vi "XXPathPlanner_ConstraintsZone_IsWithinZone.vi"(9 "T":dbl, 11 "ConstraintsZone":T1={"minPosition"=0.0, "maxPosition"=0.0, "Constraints"={"MaxVelocityMps;"=0.0, "MaxAccelerationMpsSq;"=0.0, "MaxAngularVelRadPsEc;"=0.0, "MaxAngularAccRadPSecSq"=0.0, "Exists"=FALSE, "Unlimited"=FALSE, "NominalVoltageVolts"=12.0}, "Present"=FALSE}) -> (3 "WithinZone":bool)   [LabVIEW 2019]
doc: "Get if a given waypoint relative position is within this zone\n \nInputs:\n -- ConstraintsZone -- cluster -- data structure containing zone definition. \n -- t - double - Waypoint relative position\n\nOutputs:\n -- WithinZone - boolean - True if given position is within this zone"
uses:
  TypeDef/PathPlannerConstraintsZone.ctl
  TypeDef/PathPlannerPathConstraints.ctl
  PathPlanner24.lvlib
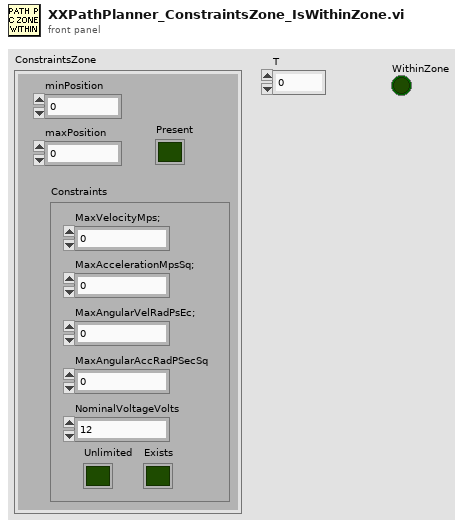
[diagram p1: front panel]
types:
  T1 = typedef "PathPlanner24.lvlib/PathPlannerConstraintsZone.ctl" = cluster{"minPosition":dbl, "maxPosition":dbl, "Constraints":T2, "Present":bool}
  T2 = typedef "PathPlanner24.lvlib/PathPlannerPathConstraints.ctl" = cluster{"MaxVelocityMps;":dbl, "MaxAccelerationMpsSq;":dbl, "MaxAngularVelRadPsEc;":dbl, "MaxAngularAccRadPSecSq":dbl, "Exists":bool, "Unlimited":bool, "NominalVoltageVolts":dbl}
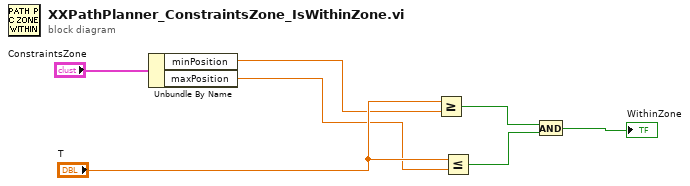
[diagram p0: block diagram]
diagram:
  n1 = Unbundle By Name("ConstraintsZone") -> ("minPosition"=w5:dbl, "maxPosition"=w4:dbl)
  n2 = Greater Or Equal?(x="T", y=w5) -> (x >= y?=w3:bool)
  n3 = Less Or Equal?(x="T", y=w4) -> (x <= y?=w2:bool)
  n4 = And(x=w3, y=w2) -> (x .and. y?=→"WithinZone":bool)
